vi "Load Config.vi"(8 "error in (no error)":errorcluster, 11 "SIM Motion Controller in":refnum<class "SIM Motion Controller.lvclass">) -> (0 "error out":errorcluster, 3 "SIM Motion Controller out":refnum<class "SIM Motion Controller.lvclass">)   [LabVIEW 2022 SP3, in "SIM Motion Controller.lvclass"]
uses:
  SIM Motion Controller.lvclass
  SIM Motion Controller.lvclass/SIM Motion Controller.ctl
  Motion Controller/Motion Controller.lvclass
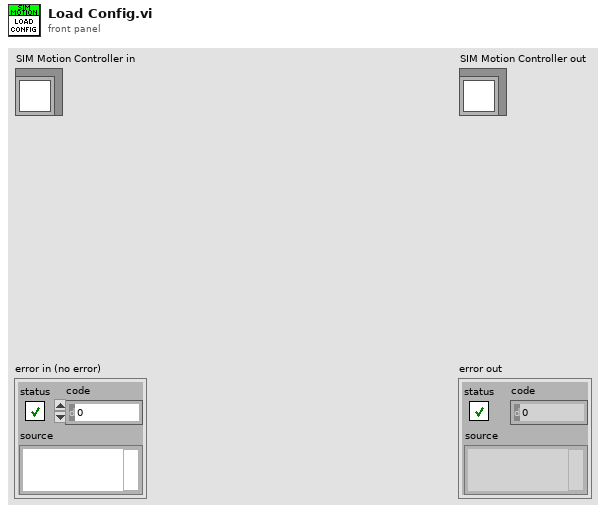
[diagram p1: front panel]
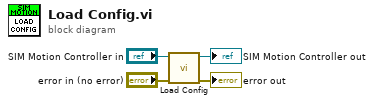
[diagram p0: block diagram]
diagram:
  n1 = call-parent "Load Config.vi"("error in (no error)"="error in (no error)", "Motion Controller in"="SIM Motion Controller in") -> ("error out"=→"error out":errorcluster, "Motion Controller out"=→"SIM Motion Controller out":refnum<class "SIM Motion Controller.lvclass">)  [unwired: 8 in]
